vi "LabVIEW Data to Python String (String).vi"(8 "error in (no error)":errorcluster, 10 "LabVIEW Data":string) -> (0 "error out":errorcluster, 2 "Python String":string)   [LabVIEW 2020, in "jki_python_data_tools.lvlib"]
doc: "Writes a value associated with key in a specified section of the configuration data identified by refnum. If \"key\" input is not specified, the name of the variant object is used as the key.\n\nFor example a Boolean named \"Enable\" with a value of TRUE would correspond to the key-value pair:\n\nEnable=TRUE"
uses:
  jki_python_data_tools.lvlib
panel:
  # "Copyright © 2003-2009 JKI. All rights reserved.\n\nAuthor: Jim Kring [jim.kring@jameskring.com]\n\nThis library is provided \"AS IS\" ,WITHOUT WARRANTIES OR \nCONDITIONS OF ANY KIND, either express or implied.\n\nJames Kring, Inc. -- http://www.jameskring.com"
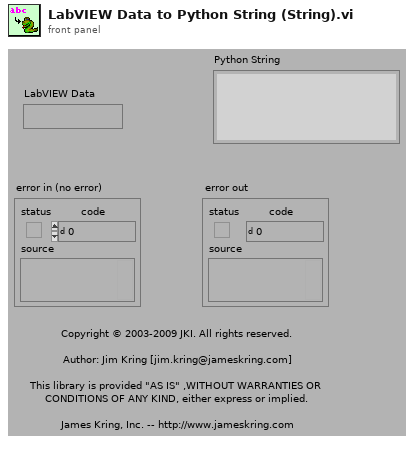
[diagram p1: front panel]
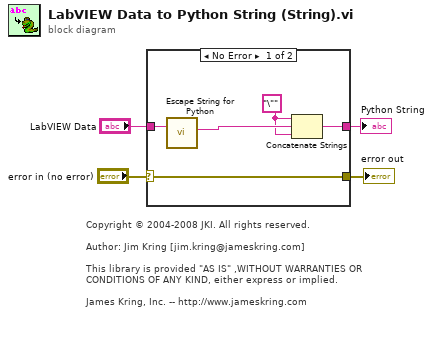
[diagram p0: block diagram]
diagram:
  # "Copyright © 2004-2008 JKI. All rights reserved.\n\nAuthor: Jim Kring [jim.kring@jameskring.com]\n\nThis library is provided \"AS IS\" ,WITHOUT WARRANTIES OR \nCONDITIONS OF ANY KIND, either express or implied.\n\nJames Kring, Inc. -- http://www.jameskring.com"
  n1 = case shown="No Error" "error in (no error)" {
    selector: "error in (no error)" -> [w5 w10]
    tunnel: "LabVIEW Data" -> [w9 w11]
    tunnel: [w6 w11] -> w3
    tunnel: [w5 w10] -> w1
    frame No Error {
      w7 = "\"" ("format string")
      n2 = call "Escape String for Python.vi"("String"=w9) -> ("Escaped Python String"=w8:string)  [unwired: 10 in]
      n3 = Concatenate Strings(w7, w8, w7) -> (w6:string)
    }
    frame Error {
    }
  }
  "error out" <- w1
  "Python String" <- w3
